vi "thermometer1_api_change_units.vi"(8 "units":T1=enum."C", 10 "target (\"thermometer1\")":string="thermometer1", 11 "sender":string) -> ()   [LabVIEW 2019]
doc: "Sends the \"unit\" msg to the <b>target</b> thermometer. Use this to change the <b>Units</b> of measurement for the targetted thermometer."
uses:
  thermometer1 support vi/thermometer1_units.ctl
  common/common data types/common_event_data.ctl
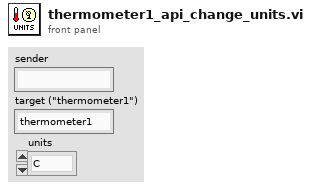
[diagram p1: front panel]
types:
  T1 = typedef "thermometer1_units.ctl" = enum16{"<select>", "C", "F", "K"}
  T2 = typedef "common_event_data.ctl" = cluster{"sender":string, "target":string, "msg":string, "data":variant}
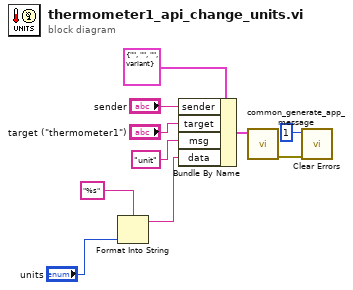
[diagram p0: block diagram]
diagram:
  n1 = Format Into String(format string="%s", "units") -> (resulting string=w5:string)  [unwired: 2 in, 1 out]
  n2 = Bundle By Name(cluster=T2 {"sender"="", "target"="", "msg"="", "data"=variant} ("event data"), "sender"="sender", "target"="target (\"thermometer1\")", "msg"="unit", "data"=w5) -> (w4:T2)
  n3 = call "common_generate_app_message.vi"("event data"=w4) -> ("error out"=w3:errorcluster)  [unwired: 10 in]
  n4 = call <vilib>:"Clear Errors.vi"("error in (no error)"=w3, "specific error code to clear (0: all)"=1) -> ()  [unwired: 4 in, 2 out]
